vi "手动启动选择对话框.vi"() -> (1 "二级进样 2":bool, 2 "确定":bool, 3 "输出簇":T1)   [LabVIEW 2016, in "PLC.lvlib"]
uses:
  PLC.lvlib
panel:
  in  "二级进样":bool
  in  "总磷":bool
  in  "测试模式":enum16{"正常测试", "集成干预"}(ring)
  in  "CODCr":bool
  in  "总氮":bool
  in  "氨氮":bool
  in  "CODmn":bool
  in  "多参数":bool
  in  "取消":bool
  in  "确定":bool
  # "请选择启动参数"
  # "请选择启动模式："
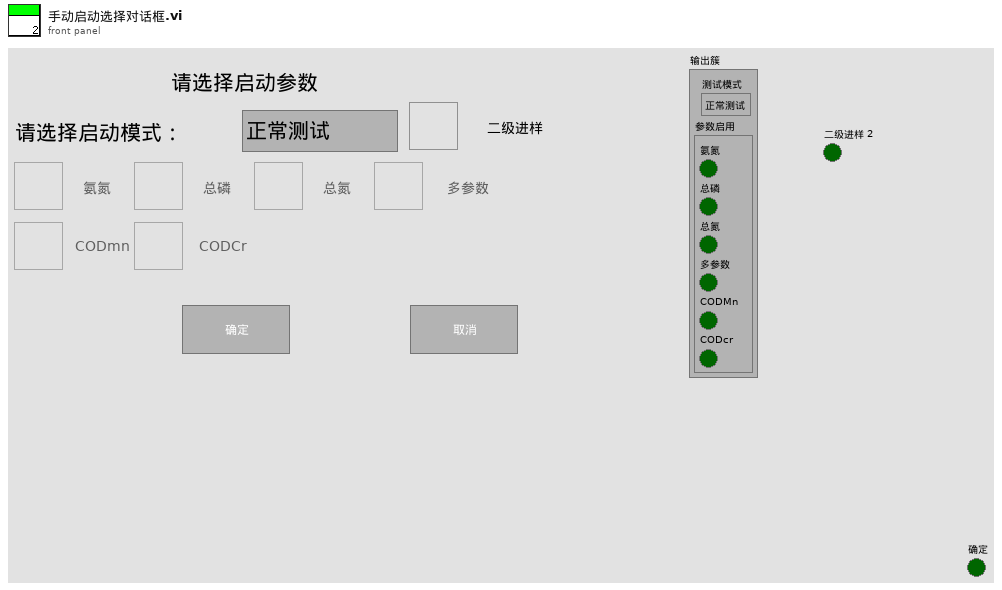
[diagram p1: front panel]
types:
  T1 = cluster{"测试模式":enum16{"正常测试", "集成干预"}, "参数启用":cluster{"氨氮":bool, "总磷":bool, "总氮":bool, "多参数":bool, "CODMn":bool, "CODcr":bool}}
  T2 = enum8{"Enabled", "Disabled", "Disabled and Grayed Out"}
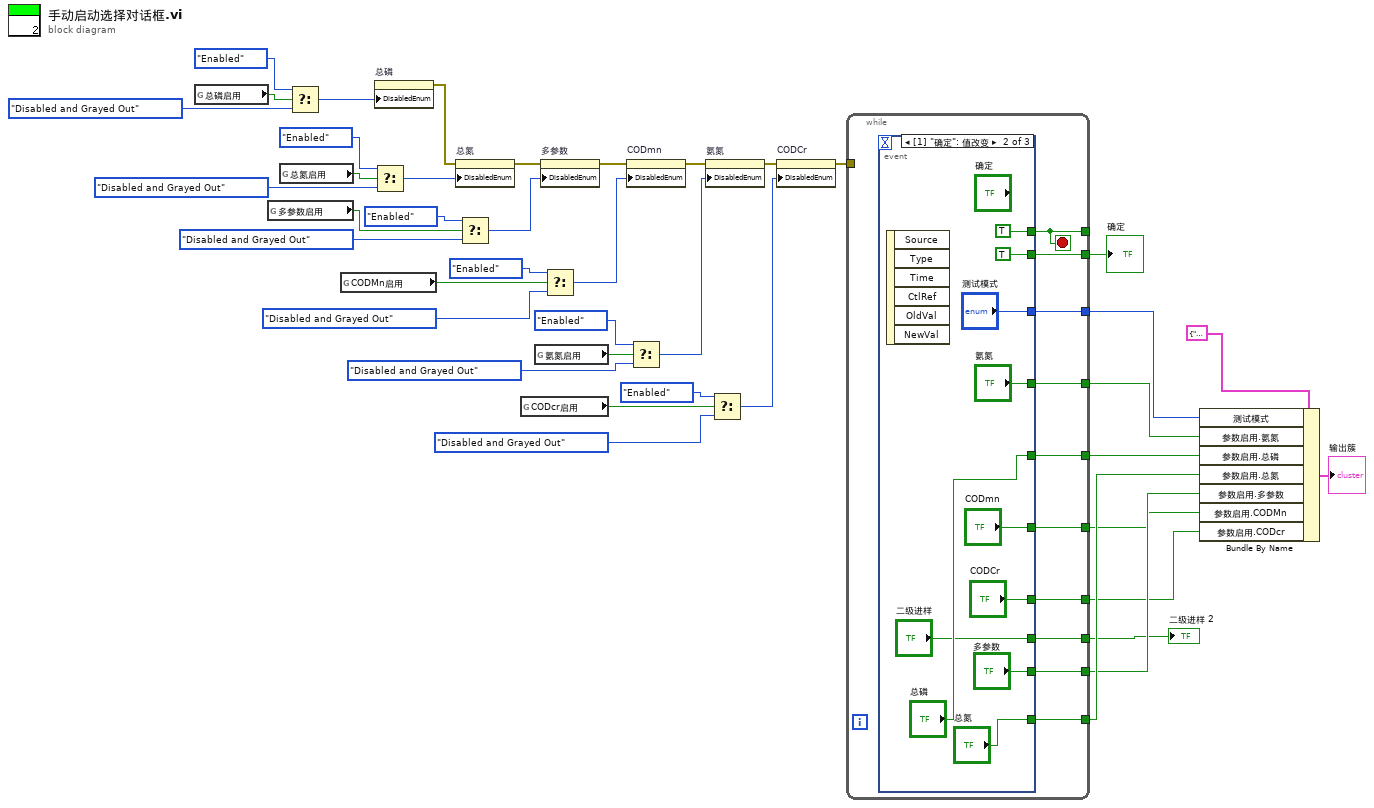
[diagram p0: block diagram]
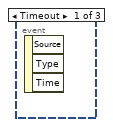
[diagram p2: hidden frame]
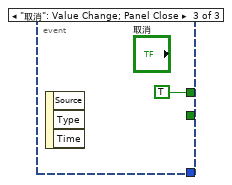
[diagram p3: hidden frame]
diagram:
  n1 = global read "系统设置全局变量.vi" "总磷启用"() -> (w9:bool)
  n2 = global read "系统设置全局变量.vi" "多参数启用"() -> (w22:bool)
  n3 = global read "系统设置全局变量.vi" "总氮启用"() -> (w40:bool)
  n4 = Select(t=T2."Enabled" ("禁用"), s=w9, f=T2."Disabled and Grayed Out" ("禁用")) -> (s? t:f=w12:T2)
  n5 = global read "系统设置全局变量.vi" "CODMn启用"() -> (w26:bool)
  n6 = property on="总磷" class="Bool (严格)"("DisabledEnum"=w12) -> (error out=w8:errorcluster)  [unwired: 2 in, 1 out]
  n7 = Select(t=T2."Enabled" ("禁用"), s=w40, f=T2."Disabled and Grayed Out" ("禁用")) -> (s? t:f=w37:T2)
  n8 = property on="总氮" class="Bool (严格)"(error in=w8, "DisabledEnum"=w37) -> (error out=w20:errorcluster)  [unwired: 1 in, 1 out]
  n9 = Select(t=T2."Enabled" ("禁用"), s=w22, f=T2."Disabled and Grayed Out" ("禁用")) -> (s? t:f=w21:T2)
  n10 = global read "系统设置全局变量.vi" "CODcr启用"() -> (w24:bool)
  n11 = global read "系统设置全局变量.vi" "氨氮启用"() -> (w28:bool)
  n12 = property on="多参数" class="Bool (严格)"(error in=w20, "DisabledEnum"=w21) -> (error out=w19:errorcluster)  [unwired: 1 in, 1 out]
  n13 = Select(t=T2."Enabled" ("禁用"), s=w26, f=T2."Disabled and Grayed Out" ("禁用")) -> (s? t:f=w25:T2)
  n14 = property on="CODmn" class="Bool (严格)"(error in=w19, "DisabledEnum"=w25) -> (error out=w18:errorcluster)  [unwired: 1 in, 1 out]
  n15 = Select(t=T2."Enabled" ("禁用"), s=w28, f=T2."Disabled and Grayed Out" ("禁用")) -> (s? t:f=w27:T2)
  n16 = property on="氨氮" class="Bool (严格)"(error in=w18, "DisabledEnum"=w27) -> (error out=w17:errorcluster)  [unwired: 1 in, 1 out]
  n17 = Select(t=T2."Enabled" ("禁用"), s=w24, f=T2."Disabled and Grayed Out" ("禁用")) -> (s? t:f=w23:T2)
  n18 = property on="CODCr" class="Bool (严格)"(error in=w17, "DisabledEnum"=w23) -> (error out=w16:errorcluster)  [unwired: 1 in, 1 out]
  n19 = while {
    tunnel: [w51] -> w5
    tunnel: [w50] -> w14
    tunnel: [w49] -> w4
    tunnel: [w48] -> _
    tunnel: [w47] -> w41
    tunnel: [w46] -> w13
    tunnel: [w45] -> w3
    tunnel: w16 -> [_]
    tunnel: [w44] -> w15
    tunnel: [w43] -> w6
    tunnel: [w42] -> w1
    stop <- w48 stop-if-true
    n20 = event shown="[1] \"确定\": 值改变" {
      selector: _ -> [_ _ _]
      dyn-events: _ -> [_ _ _]
      timeout: _ -> [_ _ _]
      tunnel: [_ TRUE TRUE] -> w48
      tunnel: [_ "多参数" _] -> w51
      tunnel: [_ "氨氮" _] -> w50
      tunnel: [_ "CODmn" _] -> w49
      tunnel: [_ TRUE _] -> w47
      tunnel: [_ "总磷" _] -> w46
      tunnel: [_ "CODCr" _] -> w45
      tunnel: [_ "测试模式" _] -> w44
      tunnel: [_ "总氮" _] -> w43
      tunnel: [_ "二级进样" _] -> w42
      event Timeout {
        n21 = event-data() -> ()  [unwired: 1 in, 3 out]
      }
      event "确定": Value Change {
        n22 = event-data() -> ()  [unwired: 1 in, 6 out]
      }
      event "取消": Value Change; Panel Close {
        n23 = event-data() -> ()  [unwired: 1 in, 3 out]
      }
    }
  }
  "确定" <- w41
  "二级进样 2" <- w1
  n24 = Bundle By Name(cluster=T1 {"测试模式"=enum."正常测试", "参数启用"={"氨氮"=FALSE, "总磷"=FALSE, "总氮"=FALSE, "多参数"=FALSE, "CODMn"=FALSE, "CODcr"=FALSE}} ("参数"), "测试模式"=w15, "参数启用.氨氮"=w14, "参数启用.总磷"=w13, "参数启用.总氮"=w6, "参数启用.多参数"=w5, "参数启用.CODMn"=w4, "参数启用.CODcr"=w3) -> (→"输出簇":T1)
